vi "Pi-Drive.vi"(6 "turbo":bool, 8 "Engage QuickTurn":bool, 9 "Turn":dbl min=-1.0 step=0.1, 10 "Throttle":dbl min=-1.0 max=1.0 step=0.1) -> (2 "Right Drive":dbl, 3 "Left Drive":dbl)   [LabVIEW 2019]
panel:
  in  "No Quickturn Min Throttle":dbl=0.4
  in  "Throttle Increase Curve":dbl=2.0
  in  "Turn Increase Curve":dbl=3.0
  out "Right Drive Chart":dbl(graph)
  out "Left Drive Chart":dbl(graph)
  in  "True - Momentum On\nFalse - Momentum Off":bool=TRUE
  in  "Momentum Gain":dbl=2.0
  in  "Throttle Deadband":dbl=0.03
  in  "Turn Deadband":dbl=0.03
  in  "Turn While Drive Gain":dbl=1.0 min=-1.0 step=0.1
  in  "QuickTurn Gain":dbl=0.3 format="%#_13g"
  out "Right Drive After Normal":dbl
  out "Left Drive After Normal":dbl
  # "Inputs"
  # "Controls"
  # "Momentum"
  # "Indicators"
  # "Outputs"
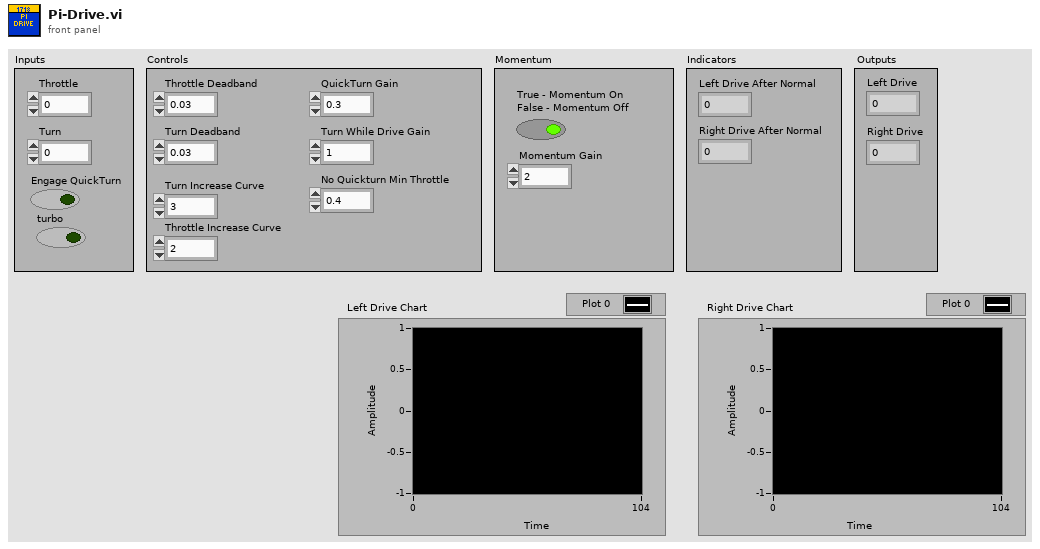
[diagram p1: front panel]
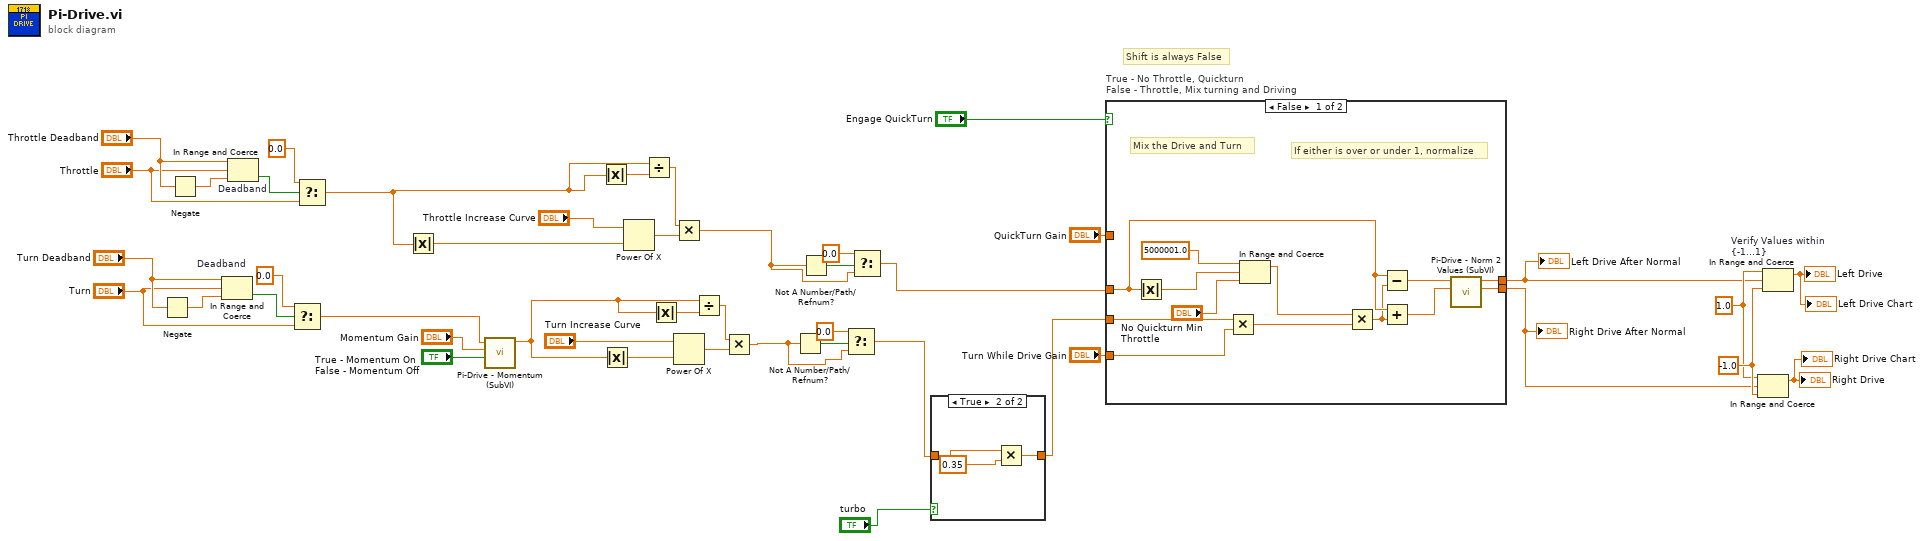
[diagram p0: block diagram]
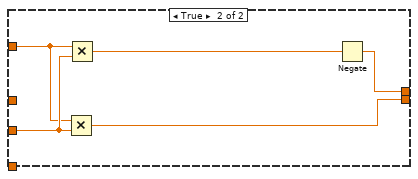
[diagram p3: hidden frame]
diagram:
  w44 = -1.0 ("lower limit")
  w43 = 1.0 ("upper limit")
  # "Shift is always False"
  n1 = Negate(x="Turn Deadband") -> (-x=w40:dbl)
  n2 = Negate(x="Throttle Deadband") -> (-x=w38:dbl)
  n3 = In Range and Coerce "Deadband"(upper limit="Turn Deadband", x="Turn", lower limit=w40) -> (In Range?=w36:bool)  [unwired: 1 out]
  n4 = In Range and Coerce "Deadband"(upper limit="Throttle Deadband", x="Throttle", lower limit=w38) -> (In Range?=w33:bool)  [unwired: 1 out]
  n5 = Select(t=0.0 ("Turn"), s=w36, f="Turn") -> (s? t:f=w30:dbl)
  n6 = Select(t=0.0 ("Turn"), s=w33, f="Throttle") -> (s? t:f=w23:dbl)
  n7 = Absolute Value(x=w23) -> (abs(x)=w24:dbl)
  n8 = call "Pi-Drive - Momentum (SubVI).vi"("True - Momentum On\nFalse - Momentum Off"="True - Momentum On\nFalse - Momentum Off", "Momentum Gain"="Momentum Gain", "Turn in"=w30) -> ("Turn out"=w14:dbl)  [unwired: 8 in]
  n9 = Absolute Value(x=w23) -> (abs(x)=w22:dbl)
  n10 = Absolute Value(x=w14) -> (abs(x)=w16:dbl)
  n11 = Power Of X(1:w24, 2:"Throttle Increase Curve") -> (0:w21:dbl)
  n12 = Divide(x=w23, y=w22) -> (x/y=w20:dbl)
  n13 = Absolute Value(x=w14) -> (abs(x)=w17:dbl)
  n14 = Multiply(x=w20, y=w21) -> (x*y=w9:dbl)
  n15 = Power Of X(1:w16, 2:"Turn Increase Curve") -> (0:w18:dbl)
  n16 = Divide(x=w14, y=w17) -> (x/y=w19:dbl)
  n17 = Multiply(x=w19, y=w18) -> (x*y=w5:dbl)
  n18 = Not A Number/Path/Refnum?(number/path/refnum=w5) -> (NaN/Path/Refnum?=w7:bool)
  n19 = Not A Number/Path/Refnum?(number/path/refnum=w9) -> (NaN/Path/Refnum?=w10:bool)
  n20 = Select(t=0.0, s=w7, f=w5) -> (s? t:f=w2:dbl)
  n21 = Select(t=0.0, s=w10, f=w9) -> (s? t:f=w8:dbl)
  n22 = case shown="True" "turbo" {
    tunnel: w2 -> [w45 w46]
    tunnel: [w45 w48] -> w1
    frame False {
    }
    frame True {
      n23 = Multiply(x=w46, y=0.35) -> (x*y=w48:dbl)
    }
  }
  n24 = case "True - No Throttle, Quickturn\nFalse - Throttle, Mix turning and Driving" shown="False" "Engage QuickTurn" {
    tunnel: w1 -> [w56 w66]
    tunnel: [w58 w62] -> w41
    tunnel: [w59 w63] -> w42
    tunnel: w8 -> [w61 _]
    tunnel: "QuickTurn Gain" -> [_ w65]
    tunnel: "Turn While Drive Gain" -> [w55 _]
    frame False {
      # "If either is over or under 1, normalize"
      # "Mix the Drive and Turn"
      n25 = Absolute Value(x=w61) -> (abs(x)=w52:dbl)
      n26 = Multiply(x=w56, y=w55) -> (x*y=w57:dbl)
      n27 = In Range and Coerce(upper limit=5000001.0, x=w52, lower limit="No Quickturn Min Throttle") -> (coerced(x)=w49:dbl)  [unwired: 1 out]
      n28 = Multiply(x=w49, y=w57) -> (x*y=w60:dbl)
      n29 = Subtract(x=w61, y=w60) -> (x-y=w54:dbl)
      n30 = Add(x=w61, y=w60) -> (x+y=w53:dbl)
      n31 = call "Pi-Drive - Norm 2 Values (SubVI).vi"("Value 2"=w53, "Value 1"=w54) -> ("Output Value 2"=w58:dbl, "Output Value 1"=w59:dbl)  [unwired: 8 in]
    }
    frame True {
      n32 = Multiply(x=w65, y=w66) -> (x*y=w62:dbl)
      n33 = Multiply(x=w65, y=w66) -> (x*y=w64:dbl)
      n34 = Negate(x=w64) -> (-x=w63:dbl)
    }
  }
  "Left Drive After Normal" <- w42
  "Right Drive After Normal" <- w41
  n35 = In Range and Coerce(upper limit=w43, x=w41, lower limit=w44) -> (coerced(x)=→"Right Drive" →"Right Drive Chart":dbl)  [unwired: 1 out]
  n36 = In Range and Coerce "Verify Values within\n{-1...1}"(upper limit=w43, x=w42, lower limit=w44) -> (coerced(x)=→"Left Drive" →"Left Drive Chart":dbl)  [unwired: 1 out]
